vi "_Start Monitor VI.vi"(8 "error in (no error)":errorcluster) -> (0 "error out":errorcluster)   [LabVIEW 2017, in "tagdb-probe-support.lvlib"]
uses:
  tagdb-probe-support.lvlib
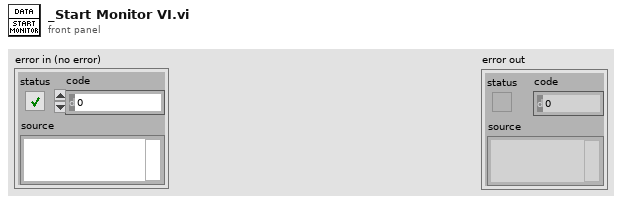
[diagram p1: front panel]
types:
  T1 = enum32{"Bad", "Idle", "Run top level", "Running"}
  T2 = enum32{"Invalid", "Standard", "Closed", "Hidden", "Minimized", "Maximized"}
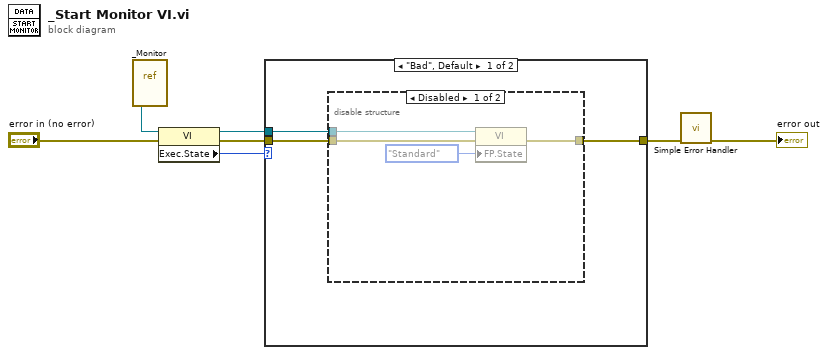
[diagram p0: block diagram]
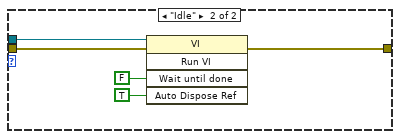
[diagram p3: hidden frame]
diagram:
  n1 = vi-ref "_Monitor.vi"() -> (w7:refnum<vi>)
  n2 = property class="VI"(reference=w7, error in="error in (no error)") -> (reference out=w4:refnum<vi>, error out=w6:errorcluster, "Exec.State"=w5:T1)
  n3 = case shown="\"Bad\", Default" w5 {
    tunnel: w6 -> [w10 w19]
    tunnel: w4 -> [w8 w20]
    tunnel: [w9 w16] -> w3
    frame "Bad", Default {
      n4 = disable-structure shown="Disabled" {
        disable-tunnel: w10 -> [w14 w15]
        disable-tunnel: [w13 w15] -> w9
        disable-tunnel: w8 -> [w12 _]
        frame Disabled {
          n5 = property class="VI"(reference=w12, error in=w14, "FP.State"=T2."Standard" ("Front Panel Window:State")) -> (error out=w13:errorcluster)  [unwired: 1 out]
        }
        frame Enabled {
        }
      }
    }
    frame "Idle" {
      n6 = invoke class="VI" method="Run VI"(reference=w20, error in=w19, "Wait until done"=FALSE ("Wait Until Done"), "Auto Dispose Ref"=TRUE ("Auto Dispose Reference")) -> (error out=w16:errorcluster)  [unwired: 1 in, 4 out]
    }
  }
  n7 = call <vilib>:"Simple Error Handler.vi"("error in (no error)"=w3) -> ("error out"=→"error out":errorcluster)  [unwired: 4 in, 4 out]
